vi "Retain All.vi"(8 "error in (no error)":errorcluster, 10 "Toggle":bool[](array[boolean]), 11 "Collection in":refnum<class "Collection.lvclass">) -> (0 "error out":errorcluster, 3 "Collection out":refnum<class "Collection.lvclass">)   [LabVIEW 2023, in "Collection.lvclass"]
uses:
  Collection.lvclass
  Readable/Readable.lvclass
  Collection.lvclass/Collection.ctl
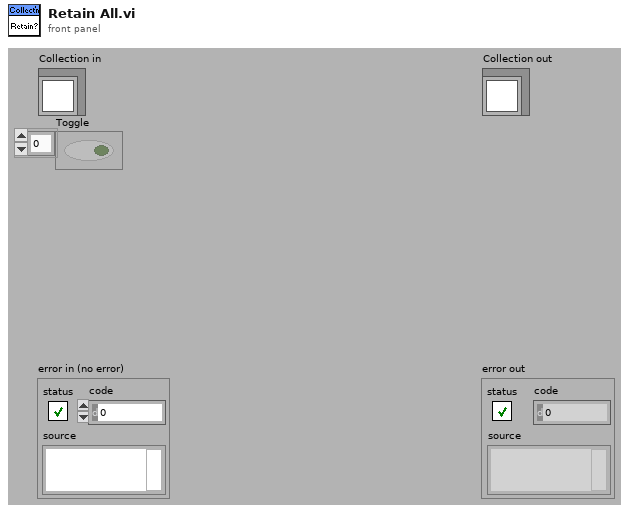
[diagram p1: front panel]
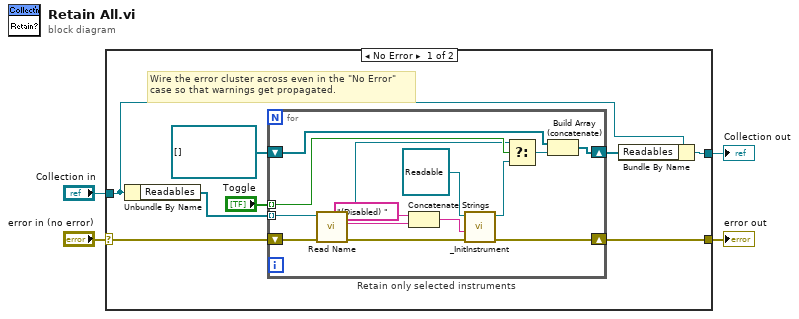
[diagram p0: block diagram]
diagram:
  n1 = case shown="No Error" "error in (no error)" {
    selector: "error in (no error)" -> [w6 w28]
    tunnel: [w5 w28] -> w3
    tunnel: [w9 w27] -> w1
    tunnel: "Collection in" -> [w11 w27]
    frame No Error {
      # "Wire the error cluster across even in the \"No Error\"\ncase so that warnings get propagated."
      n2 = Unbundle By Name(w11) -> ("Readables"=w10:refnum<class "Readable.lvclass">[])
      n3 = for "Retain only selected instruments" {
        tunnel: w10 -> [w24] mode=indexing
        shift-right: [w26] -> w8
        shift-left: refnum<class "Readable.lvclass">[] [] -> [w13]
        tunnel: "Toggle" -> [w22] mode=indexing
        shift-right: [w14] -> w5
        shift-left: w6 -> [w15]
        n4 = call-dynamic "Read Name.vi"("error in (no error)"=w15, "Instrument.lvclass in"=w24) -> ("error out"=w16:errorcluster, "Name"=w18:string, "Instrument.lvclass out"=w21:refnum<class "Readable.lvclass">)  [unwired: 7 out]
        n5 = Concatenate Strings("(Disabled) " ("Name"), w18) -> (w17:string)
        n6 = call-dynamic "_InitInstrument.vi"("error in (no error)"=w16, "Name"=w17, "Instrument in"=refnum<class "Readable.lvclass"> refnum ("Lockin SR830 out")) -> ("error out"=w14:errorcluster, "Instrument out"=w20:refnum<class "Readable.lvclass">)  [unwired: 3 in, 4 out]
        n7 = Select(t=w21, s=w22, f=w20) -> (s? t:f=w23:refnum<class "Readable.lvclass">)
        n8 = Build Array (concatenate)(w13, w23) -> (w26:refnum<class "Readable.lvclass">[])
      }
      n9 = Bundle By Name(cluster=w11, "Readables"=w8) -> (w9:refnum<class "Collection.lvclass">)
    }
    frame Error {
    }
  }
  "error out" <- w3
  "Collection out" <- w1
